vi "Vibe_SIMULINK.vi"(5 "Brenndauer":dbl, 7 "Iterationsschritte":i32, 8 "dt":dbl, 9 "C2H2 [mol]":dbl, 10 "CH4 [mol]":dbl, 11 "H2 [mol]":dbl) -> (2 "Aktuelle Zeit":dbl, 3 "Array":dbl[](array[numeric]))   [LabVIEW 2009]
uses:
  <vilib>/Analysis/NI_AALBase.lvlib
  <vilib>/Analysis/baseanly.llb/Real Dot Product.vi
panel:
  out "Signalverlaufsgraph":dbl[](graph)
  out "Max. Wert":dbl
  in  "m":dbl
  in  "a":dbl
  in  "Molare Heizwerte [kJ/mol]":dbl[](array[numeric]) min=1255.6 max=1255.6
  # "H2"
  # "CH4"
  # "C2H2"
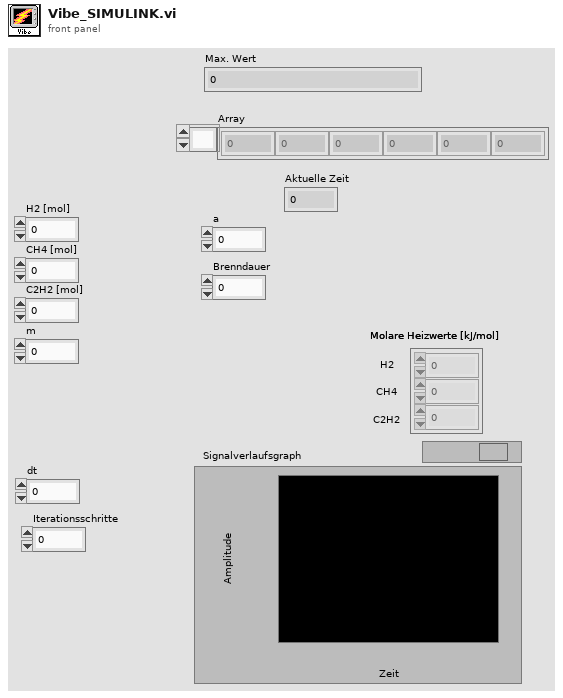
[diagram p1: front panel]
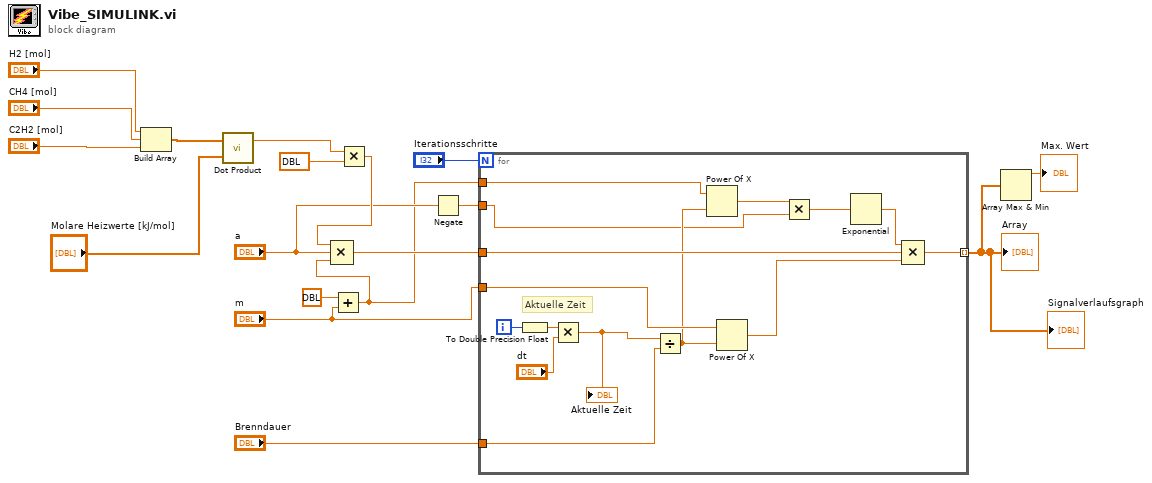
[diagram p0: block diagram]
diagram:
  n1 = Build Array("H2 [mol]", "CH4 [mol]", "C2H2 [mol]") -> (w12:dbl[])
  n2 = call-poly <vilib>:"Dot Product.vi"("Y Vector"="Molare Heizwerte [kJ/mol]", "X Vector"=w12) -> ("X * Y"=w11:dbl)  [unwired: 1 out]
  n3 = Add(x=dbl ?, y="m") -> (x+y=w3:dbl)
  n4 = Multiply(x=w11, y=dbl ? ("Summe")) -> (x*y=w10:dbl)
  n5 = Compound Arithmetic op=MULTIPLY(w10, "a", w3) -> (w9:dbl)
  n6 = Negate(x="a") -> (-x=w4:dbl)
  n7 = for {
    N: "Iterationsschritte" -> [_]
    tunnel: w9 -> [w28]
    tunnel: "Brenndauer" -> [w30]
    tunnel: "m" -> [w29]
    tunnel: w4 -> [w22]
    tunnel: w3 -> [w26]
    tunnel: [w20] -> w1 mode=indexing
    i -> [w32]
    # "Aktuelle Zeit"
    n8 = To Double Precision Float(number=w32) -> (double precision float=w31:dbl)
    n9 = Multiply(x=w31, y="dt") -> (x*y=w19:dbl)
    "Aktuelle Zeit" <- w19
    n10 = Divide(x=w19, y=w30) -> (x/y=w24:dbl)
    n11 = Power Of X(1:w24, 2:w26) -> (0:w23:dbl)
    n12 = Power Of X(1:w24, 2:w29) -> (0:w27:dbl)
    n13 = Multiply(x=w23, y=w22) -> (x*y=w21:dbl)
    n14 = Exponential(1:w21) -> (0:w25:dbl)
    n15 = Compound Arithmetic op=MULTIPLY(w25, w28, w27) -> (w20:dbl)
  }
  "Array" <- w1
  "Signalverlaufsgraph" <- w1
  n16 = Array Max & Min(array=w1) -> (max value=→"Max. Wert":dbl)  [unwired: 3 out]
